vi "Write temporary data.vi"(7 "Application path":path, 8 "Error In":errorcluster, 9 "Humidity":dbl, 10 "Temperature":dbl, 11 "MAC address":string) -> (0 "Error Out":errorcluster, 3 "Result":string)   [LabVIEW 2016]
uses:
  <vilib>/Utility/file.llb/Read Delimited Spreadsheet (DBL).vi
  <vilib>/Utility/file.llb/Write Delimited Spreadsheet (DBL).vi
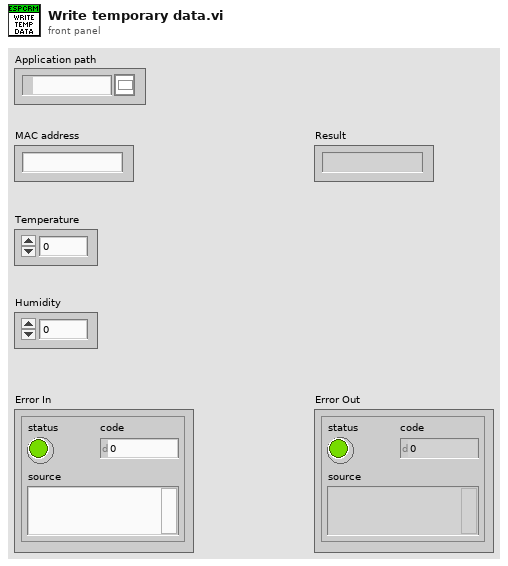
[diagram p1: front panel]
types:
  T1 = enum16{"open", "replace", "create", "open or create", "replace or create", "replace or create with confirmation"}
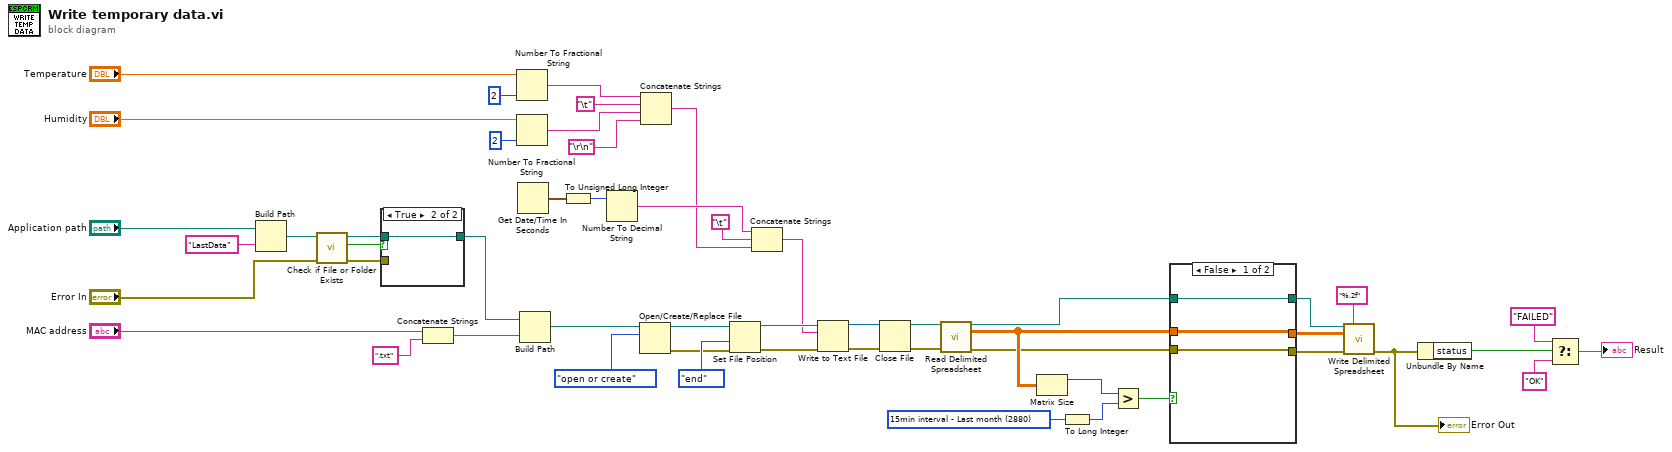
[diagram p0: block diagram]
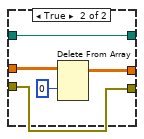
[diagram p2: hidden frame]
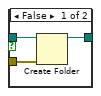
[diagram p3: hidden frame]
diagram:
  w12 = u16 2880 items=["5min interval - Last week"=2016, "5min interval - Last month"=8640, "10min interval - Last week"=1008, "10min interval - Last month"=4320, "15min interval - Last week"=672, "15min interval - Last month"=2880]
  n1 = Build Path(base path="Application path", name or relative path="LastData") -> (appended path=w48:path)
  n2 = call <vilib>:"Check if File or Folder Exists.vi"("error in (no error)"="Error In", "path"=w48) -> ("error out"=w47:errorcluster, "file or folder exists?"=w45:bool, "dup path"=w46:path)  [unwired: 7 in]
  n3 = case shown="True" w45 {
    tunnel: w47 -> [w55 _]
    tunnel: w46 -> [w54 w56]
    tunnel: [w53 w56] -> w13
    frame False {
      n4 = Create Folder(path (use dialog)=w54, error in=w55) -> (created path=w53:path)  [unwired: 1 in, 2 out]
    }
    frame True {
    }
  }
  n5 = Concatenate Strings("MAC address", ".txt" ("string")) -> (w43:string)
  n6 = Number To Fractional String(number="Temperature", precision (6)=i16 2) -> (F-format string=w52:string)  [unwired: 2 in]
  n7 = Number To Fractional String(number="Humidity", precision (6)=i16 2) -> (F-format string=w51:string)  [unwired: 2 in]
  n8 = Get Date/Time In Seconds() -> (seconds since 1Jan1904=w35:timestamp)
  n9 = Build Path(base path=w13, name or relative path=w43) -> (appended path=w36:path)
  n10 = To Unsigned Long Integer(number=w35) -> (unsigned 32bit integer=w30:u32)
  n11 = Number To Decimal String(number=w30) -> (decimal integer string=w33:string)  [unwired: 1 in]
  n12 = Open/Create/Replace File(file path (use dialog)=w36, operation (0:open)=T1."open or create") -> (refnum out=w41:refnum<file>, error out=w39:errorcluster)  [unwired: 4 in, 1 out]
  n13 = Concatenate Strings(w52, "\t", w51, "\r\n") -> (w32:string)
  n14 = Set File Position(refnum=w41, from (0:start)=enum16{"start", "end", "current"}."end", error in=w39) -> (refnum out=w37:refnum<file>, error out=w38:errorcluster)  [unwired: 1 in]
  n15 = Concatenate Strings(w33, "\t", w32) -> (w31:string)
  n16 = Write to Text File(file (use dialog)=w37, text=w31, error in=w38) -> (refnum out=w29:refnum<file>, error out=w28:errorcluster)  [unwired: 1 in, 1 out]
  n17 = Close File(refnum=w29, error in=w28) -> (path=w19:path, error out=w18:errorcluster)
  n18 = call-poly <vilib>:"Read Delimited Spreadsheet.vi"("file path (dialog if empty)"=w19, "error in (no error)"=w18) -> ("new file path (Not A Path if cancelled)"=w22:path, "all rows"=w24:dbl[][], "error out"=w20:errorcluster)  [unwired: 8 in, 3 out]
  n19 = Matrix Size(0:w24) -> (1:w27:i32)  [unwired: 1 out]
  n20 = To Long Integer(number=w12) -> (32bit integer=w11:i32)
  n21 = Greater?(x=w27, y=w11) -> (0:w26:bool)
  n22 = case shown="False" w26 {
    tunnel: w24 -> [w59 w64]
    tunnel: [w59 w62] -> w25
    tunnel: [w58 w61] -> w23
    tunnel: w22 -> [w58 w61]
    tunnel: [w57 w60] -> w21
    tunnel: w20 -> [w57 w60]
    frame False {
    }
    frame True {
      n23 = Delete From Array(array=w64, index (row)=0) -> (array with subset deleted=w62:dbl[][])  [unwired: 2 in, 1 out]
    }
  }
  n24 = call-poly <vilib>:"Write Delimited Spreadsheet.vi"("file path (dialog if empty)"=w23, "format (%.3f)"="%.2f", "2D data"=w25, "error in (no error)"=w21) -> ("error out"=w6:errorcluster)  [unwired: 10 in, 1 out]
  "Error Out" <- w6
  n25 = Unbundle By Name(w6) -> ("status"=w5:bool)
  n26 = Select(t="FAILED", s=w5, f="OK") -> (s? t:f=→"Result":string)
